vi "Teleop.vi"(10 "Match Info":T1={"Autonomous Elapsed Seconds"=0.0, "TeleOp Elapsed Seconds"=0.0, "Disabled Elapsed Seconds"=0.0, "Visited Autonomous"=FALSE, "Visited TeleOp"=FALSE, "Visited Disabled"=FALSE, "Autonomous Settings"={"Autonomous Style"=enum."Independent", "VI Refnum"=refnum}}, 11 "Call Context":T2) -> ()   [LabVIEW 2023]
doc: "This VI is called for each TeleOp packet received from the DS where the robot is not disabled. It is often used to read from the joysticks and update I/O or to update setpoints for timed control loops. It should complete and return within 20 milliseconds or it may miss DS packets."
uses:
  <vilib>/Rock Robotics/WPI/DriverStation/WPI_DriverStationDerivedRobotMode.ctl
  <vilib>/Rock Robotics/WPI/DriverStation/WPI_DriverStationMatch Info.ctl
  <vilib>/Rock Robotics/WPI/ThirdParty/Phoenix-LabVIEW/Motor Controller/Controls/CTRE_Phoenix_MotorControl_ControlMode.ctl
  <vilib>/Rock Robotics/WPI/Solenoid/WPI_SolenoidValue.ctl
  <vilib>/Rock Robotics/Network Tables/NT Read Boolean.vi
  <vilib>/Rock Robotics/Network Tables/NT Read Number.vi
  <vilib>/Rock Robotics/WPI/Utilities/WPI_GetSetVariantRefNum.vi
  <vilib>/Rock Robotics/Network Tables/NT Write Boolean Array.vi
  <vilib>/Rock Robotics/Network Tables/NT Write Numeric Array.vi
  Robot Global Data.vi
  <vilib>/Rock Robotics/WPI/ThirdParty/Phoenix-LabVIEW/Motor Controller/Get/CTRE_Phoenix_MotorController_GetSelectedSensorData.vi
  <vilib>/Rock Robotics/WPI/Solenoid/WPI_SolenoidSetEnum.vi
  <vilib>/Rock Robotics/WPI/ThirdParty/Phoenix-LabVIEW/Pigeon IMU/CTRE_PigeonIMU_GetAccumGyro.vi
  <vilib>/Rock Robotics/Network Tables/NT Write Number.vi
panel:
  out "Not Indexing and intaking":bool=TRUE
  out "Left Motor Encoder":i32
  out "Intake Output":dbl
  out "Sample Slider 0":dbl(slide) scale=0.0..5.0
  out "Sample Boolean 1":bool
  out "Sample Boolean 0":bool
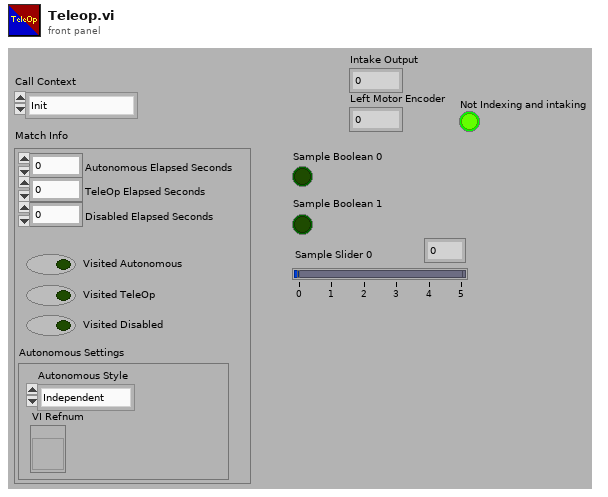
[diagram p1: front panel]
types:
  T1 = typedef "WPI_DriverStationMatch Info.ctl" = cluster{"Autonomous Elapsed Seconds":dbl, "TeleOp Elapsed Seconds":dbl, "Disabled Elapsed Seconds":dbl, "Visited Autonomous":bool, "Visited TeleOp":bool, "Visited Disabled":bool, "Autonomous Settings":cluster{"Autonomous Style":enum16{"Iterative", "Independent"}, "VI Refnum":refnum<vi>}}
  T2 = typedef "WPI_DriverStationDerivedRobotMode.ctl" = enum16{"Init", "Execute", "Stop"}
  T3 = typedef "WPI_SolenoidValue.ctl" = enum16{"Off", "On", "Forward", "Reverse"}
  T4 = typedef "CTRE_Phoenix_MotorControl_ControlMode.ctl" = u16
  T5 = typedef "WPI_JoystickDevRef.ctl" = cluster{"Device":T6}
  T6 = typedef "WPI_JoystickDeviceEnum.ctl" = enum16{"USB 0", "USB 1", "USB 2", "USB 3", "USB 4", "USB 5"}
  T7 = typedef "WPI_MotorControlDeviceRef.ctl" = cluster{"DeviceStatus":errorcluster, "Type":T8, "PWM":cluster{"PWM Channel":T9, "DeadBand":T10}, "CAN":cluster{"Device Number":u8, "SetOutput VI Ref":variant, "GetOutput VI Ref":variant, "Enable VI Ref":variant, "Disable VI Ref":variant, "Data":variant}, "Invert":bool, "DIO PWM":cluster{"PWM \"Enable\" Channel":T9, "DIOChannel":T11, "PWM Rate":dbl}}
  T8 = typedef "WPI_MotorControlType.ctl" = enum16{"PWM", "CAN", "DIO PWM"}
  T9 = typedef "FPGA_DIOPWMChannel.ctl" = enum8{"PWM 0", "PWM 1", "PWM 2", "PWM 3", "PWM 4", "PWM 5", "PWM 6", "PWM 7", "PWM 8", "PWM 9", "PWM MXP 0", "PWM MXP 1", "PWM MXP 2", "PWM MXP 3", "PWM MXP 4", "PWM MXP 5", "PWM MXP 6", "PWM MXP 7", "PWM MXP 8", "PWM MXP 9", "Invalid"}
  T10 = typedef "WPI_PWMDeadband.ctl" = cluster{"Name":string, "maxPositivePwm":i32, "minPositivePwm":i32, "centerPwm":i32, "maxNegativePwm":i32, "minNegativePwm":i32, "angularRange":u16}
  T11 = typedef "FPGA_DIOChannel.ctl" = enum8{"DIO 0", "DIO 1", "DIO 2", "DIO 3", "DIO 4", "DIO 5", "DIO 6", "DIO 7", "DIO 8", "DIO 9", "DIO MXP 0", "DIO MXP 1", "DIO MXP 2", "DIO MXP 3", "DIO MXP 4", "DIO MXP 5", "DIO MXP 6", "DIO MXP 7", "DIO MXP 8", "DIO MXP 9", "DIO MXP 10", "DIO MXP 11", "DIO MXP 12", "DIO MXP 13", "DIO MXP 14", "DIO MXP 15", "SPI Port CS1", "SPI Port CS2", "SPI Port CS3", "SPI Port MISO", "SPI Port MOSI", "Invalid"}
  T12 = typedef "WPI_RobotDriveDevRef.ctl" = cluster{"DevStatus":errorcluster, "Motors[]":T7[], "Square Inputs":bool, "Max Output":dbl}
  T13 = typedef "WPI_SolenoidDevRef.ctl" = cluster{"DevStatus":errorcluster, "Pneumatics Control Module":u8, "Forward Solenoid Channel":T14, "Reverse Solenoid Channel":T14}
  T14 = typedef "WPI_SolenoidChannel.ctl" = enum8{"Solenoid 0", "Solenoid 1", "Solenoid 2", "Solenoid 3", "Solenoid 4", "Solenoid 5", "Solenoid 6", "Solenoid 7", "Solenoid 8", "Solenoid 9", "Solenoid 10", "Solenoid 11", "Solenoid 12", "Solenoid 13", "Solenoid 14", "Solenoid 15", "Invalid"}
  T15 = typedef "WPI_ServoDeviceRef.ctl" = cluster{"DeviceStatus":errorcluster, "PWM Channel":T9, "DeadBand":T10}
  T16 = typedef "CTRE_PigeonIMU_DeviceRef.ctl" = cluster{"DeviceStatus":errorcluster, "Device Number":u8, "Type":T17, "Device ID":u32, "Handle":u64, "UsageFrame":u32, "Library Path":path}
  T17 = typedef "CTRE_PigeonIMU_ConnectionType.ctl" = u32
  T18 = typedef "WPI_SwitchDevRef.ctl" = cluster{"DevStatus":errorcluster, "DIO Channel":T11, "CntIndex":T19, "Normally Closed":bool}
  T19 = typedef "FPGA_CounterCtrSystemIndex.ctl" = enum8{"Ctr 0", "Ctr 1", "Ctr 2", "Ctr 3", "Ctr 4", "Ctr 5", "Ctr 6", "Ctr 7", "Invalid"}
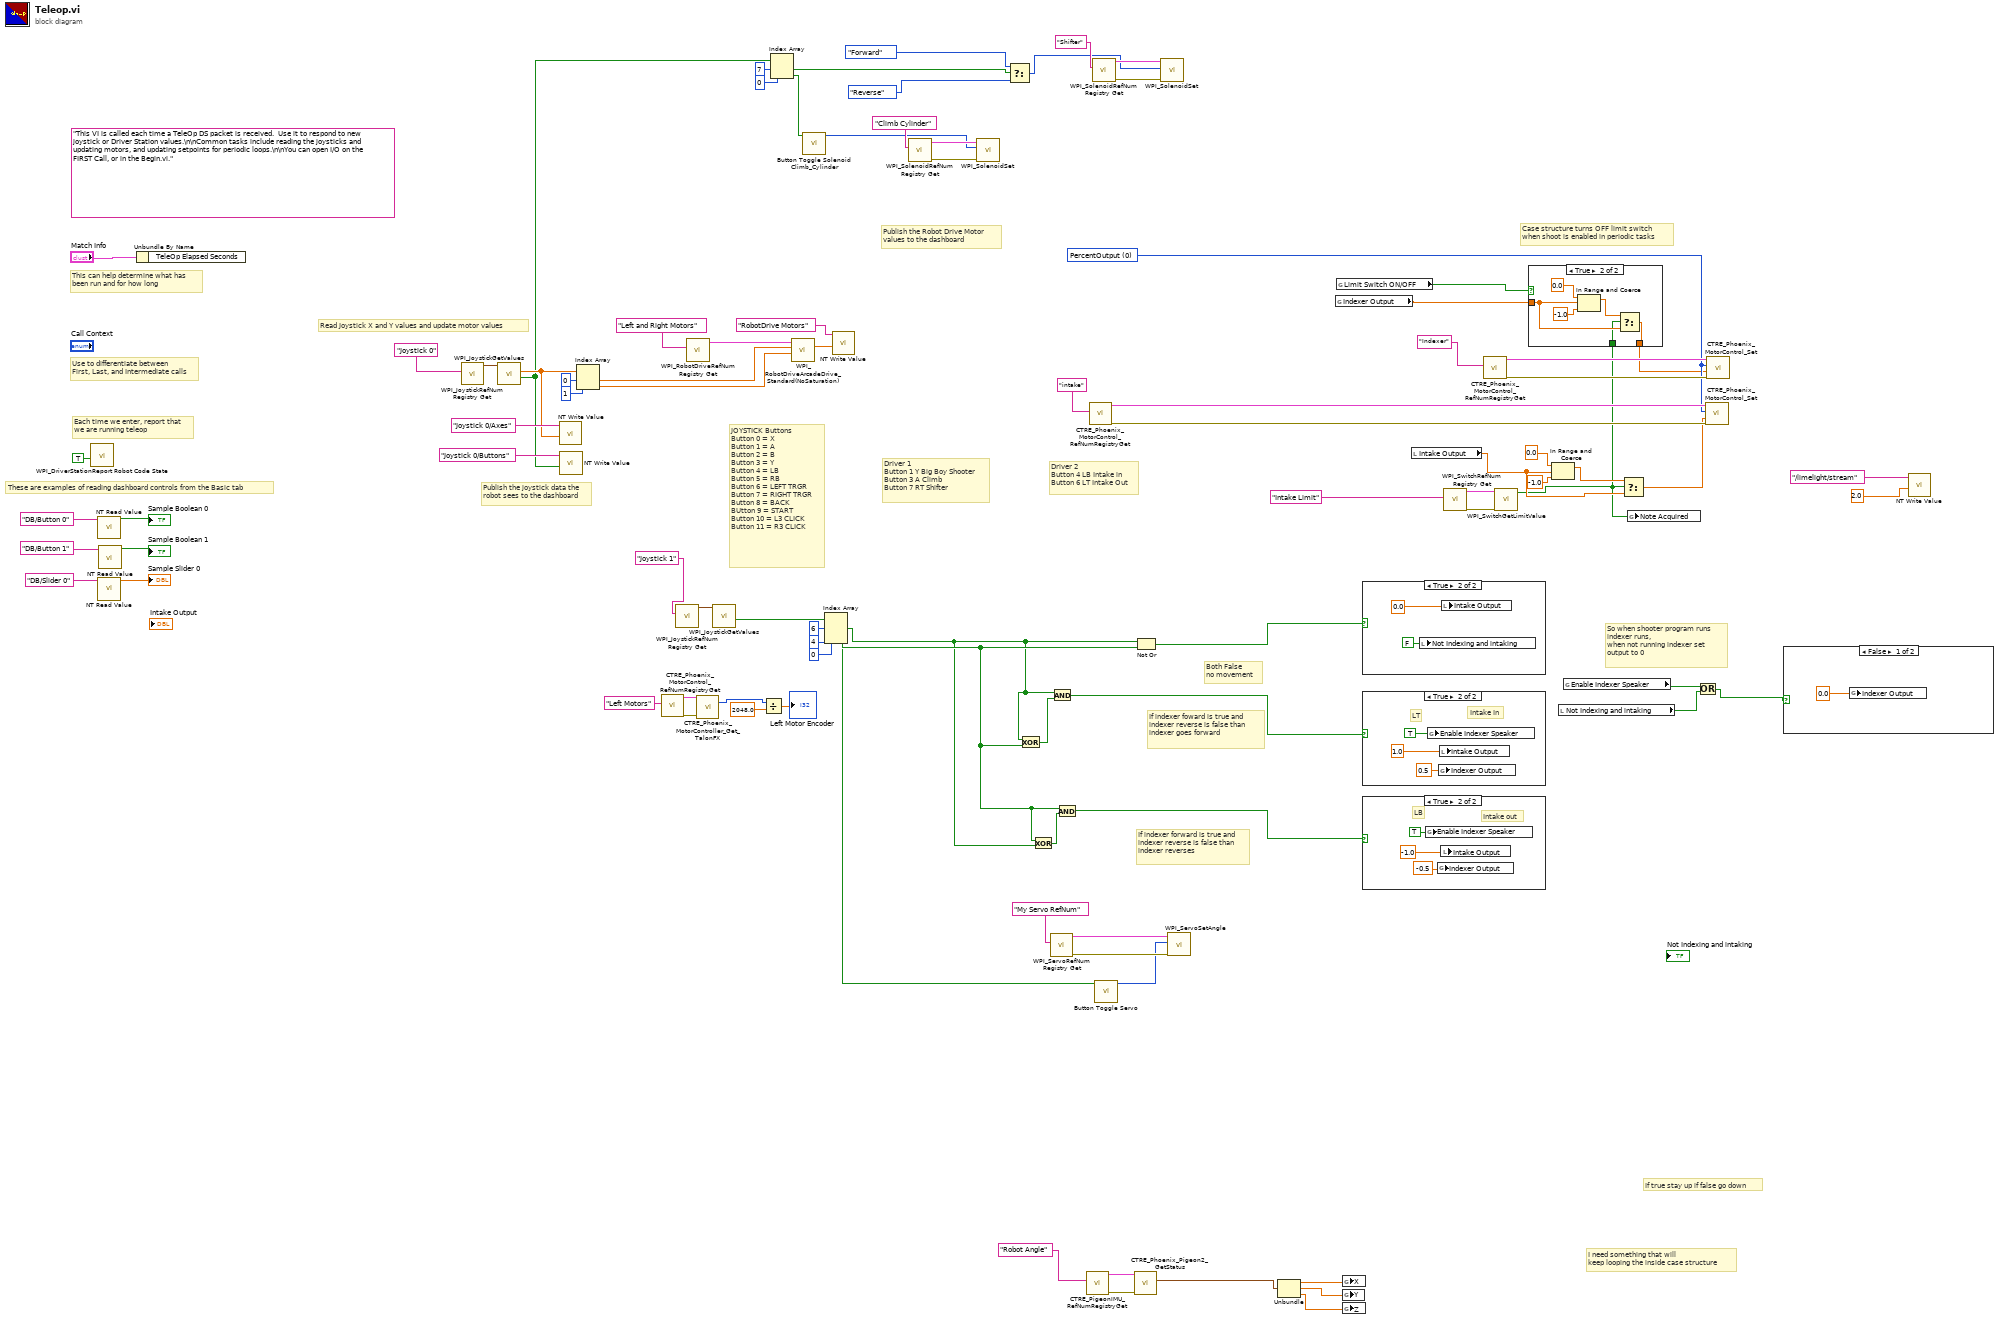
[diagram p0: block diagram]
diagram:
  w59 = T4 0 items=["PercentOutput"=0, "Position"=1, "Velocity"=2, "Current"=3, "Follower"=5, "MotionProfile"=6, "MotionMagic"=7, "MotionProfileArc"=10, "Disabled"=15] ("Control Mode")
  (unwired) "This VI is called each time a TeleOp DS packet is received.  Use it to respond to new joystick or Driver Station values.\n\nCommon tasks include reading the joysticks and updating motors, and updating setpoints for periodic loops.\n\nYou can open I/O on the FIRST Call, or in the Begin.vi."
  # "Driver 2\nButton 4 LB Intake in\nButton 6 LT Intake Out"
  # "Driver 1\nButton 1 Y Big Boy Shooter\nButton 3 A Climb\nButton 7 RT Shifter"
  # "I need something that will\nkeep looping the inside case structure"
  # "If true stay up if false go down"
  # "So when shooter program runs\nindexer runs,\nwhen not running indexer set\noutput to 0"
  # "Case structure turns OFF limit switch\nwhen shoot is enabled in periodic tasks"
  # "If indexer foward is true and\nindexer reverse is false than \nindexer goes forward"
  # "Both False\nno movement"
  # "If indexer forward is true and\nindexer reverse is false than \nindexer reverses"
  # "JOYSTICK Buttons\nButton 0 = X\nButton 1 = A\nButton 2 = B\nButton 3 = Y\nButton 4 = LB \nButton 5 = RB\nButton 6 = LEFT TRGR \nButton 7 = RIGHT TRGR \nButton 8 = BACK\nBUtton 9 = START\nButton 10 = L3 CLICK\nButton 11 = R3 CLICK"
  # "Publish the Robot Drive Motor\nvalues to the dashboard"
  # "Publish the joystick data the\nrobot sees to the dashboard"
  # "Read Joystick X and Y values and update motor values"
  # "These are examples of reading dashboard controls from the Basic tab"
  # "Each time we enter, report that\nwe are running teleop"
  # "Use to differentiate between\nFirst, Last, and Intermediate calls"
  # "This can help determine what has\nbeen run and for how long"
  n1 = call <vilib>:"WPI_DriverStationReport Robot Code State.vi"("TeleOp"=TRUE ("Autonomous")) -> ()  [unwired: 10 in, 1 out]
  n2 = call-poly <vilib>:"NT Read Value.vi"("name"="DB/Button 0" ("refnum name")) -> ("value"=→"Sample Boolean 0":bool)  [unwired: 8 in, 2 out]
  n3 = call-poly <vilib>:"NT Read Value.vi"("name"="DB/Slider 0" ("refnum name")) -> ("value"=→"Sample Slider 0":dbl)  [unwired: 8 in, 2 out]
  n4 = call-poly <vilib>:"NT Read Value.vi"("name"="DB/Button 1" ("refnum name")) -> ("value"=→"Sample Boolean 1":bool)  [unwired: 8 in, 2 out]
  n5 = Unbundle By Name("Match Info") -> ()  [unwired: 1 out]
  n6 = call <vilib>:"WPI_JoystickRefNum Registry Get.vi"("refnum name"="Joystick 0") -> ("JoystickDevRef"=w82:T5)  [unwired: 1 in, 9 out]
  n7 = call <vilib>:"WPI_JoystickGetValues.vi"("JoystickDevRef"=w82) -> ("Buttons"=w20:bool[], "Axes"=w79:dbl[])  [unwired: 6 in, 3 out]
  n8 = call-poly <vilib>:"NT Write Value.vi"("value"=w79, "name"="Joystick 0/Axes" ("Name")) -> ()  [unwired: 9 in, 1 out]
  n9 = call-poly <vilib>:"NT Write Value.vi"("value"=w20, "name"="Joystick 0/Buttons" ("Name")) -> ()  [unwired: 9 in, 1 out]
  n10 = Index Array(array=w79, index #1=0 ("index"), index #2=1 ("index")) -> (element #1=w73:dbl, element #2=w72:dbl)
  n11 = call <vilib>:"CTRE_Phoenix_MotorControl_RefNumRegistryGet.vi"("refnum name"="Left Motors") -> ("error out"=w47:errorcluster, "PhoenixMotorControlDevRef"=w48:T7)  [unwired: 9 in]
  n12 = call <vilib>:"WPI_JoystickRefNum Registry Get.vi"("refnum name"="Joystick 1") -> ("JoystickDevRef"=w18:T5)  [unwired: 1 in, 9 out]
  n13 = call <vilib>:"WPI_RobotDriveRefNum Registry Get.vi"("refnum name"="Left and Right Motors") -> ("RobotDriveDevRef"=w76:T12)  [unwired: 1 in, 9 out]
  n14 = call-poly <vilib>:"CTRE_Phoenix_MotorController_Get_TalonFX.vi"("PhoenixMotorControlDevRef"=w48, "error in"=w47) -> ("Position (Raw Sensor Units)"=w44:i32)  [unwired: 10 in, 3 out]
  n15 = call <vilib>:"WPI_JoystickGetValues.vi"("JoystickDevRef"=w18) -> ("Buttons"=w19:bool[])  [unwired: 6 in, 4 out]
  n16 = Divide(x=w44, y=2048.0) -> (x/y=→"Left Motor Encoder":dbl)
  n17 = Index Array(array=w20, index #1=7 ("index"), index #2=0 ("index")) -> (element #1=w33:bool, element #2=w31:bool)
  n18 = call <vilib>:"WPI_RobotDriveArcadeDrive_Standard(NoSaturation).vi"("Y axis value"=w72, "X axis value"=w73, "RobotDriveDevRef"=w76) -> ("Motor Values"=w75:dbl[])  [unwired: 1 in, 7 out]
  n19 = call "Button Toggle Solenoid Climb_Cylinder.vi"("Button A"=w31) -> ("Climb_Cylinder_Value"=w32:T3)  [unwired: 10 in]
  n20 = Index Array(array=w19, index #1=6 ("index"), index #2=4 ("index"), index #3=0 ("index")) -> (element #1=w13:bool, element #2=w14:bool, element #3=w6:bool)
  n21 = call-poly <vilib>:"NT Write Value.vi"("value"=w75, "name"="RobotDrive Motors" ("Name")) -> ()  [unwired: 9 in, 1 out]
  n22 = call <vilib>:"WPI_SolenoidRefNum Registry Get.vi"("refnum name"="Climb Cylinder") -> ("error out"=w36:errorcluster, "SolenoidDevRef"=w37:T13)  [unwired: 9 in]
  n23 = call-poly <vilib>:"WPI_SolenoidSet.vi"("error in (no error)"=w36, "Value"=w32, "SolenoidDevRef"=w37) -> ()  [unwired: 7 in, 2 out]
  n24 = Select(t=WPI_SolenoidValue."Forward" ("Value"), s=w33, f=WPI_SolenoidValue."Reverse" ("Value")) -> (s? t:f=w40:T3)
  n25 = Exclusive Or(1:w14, 2:w13) -> (0:w69:bool)
  n26 = Exclusive Or(1:w13, 2:w14) -> (0:w68:bool)
  n27 = call <vilib>:"WPI_ServoRefNum Registry Get.vi"("refnum name"="My Servo RefNum") -> ("error out"=w9:errorcluster, "ServoDeviceRef"=w8:T15)  [unwired: 9 in]
  n28 = And(x=w13, y=w69) -> (x .and. y?=w67:bool)
  n29 = And(x=w14, y=w68) -> (x .and. y?=w66:bool)
  n30 = call <vilib>:"CTRE_PigeonIMU_RefNumRegistryGet.vi"("refnum name"="Robot Angle") -> ("error out"=w28:errorcluster, "PigeonIMUDevRef"=w27:T16)  [unwired: 9 in]
  n31 = call <vilib>:"CTRE_Phoenix_MotorControl_RefNumRegistryGet.vi"("refnum name"="intake") -> ("error out"=w63:errorcluster, "PhoenixMotorControlDevRef"=w64:T7)  [unwired: 9 in]
  n32 = call <vilib>:"WPI_SolenoidRefNum Registry Get.vi"("refnum name"="Shifter") -> ("error out"=w42:errorcluster, "SolenoidDevRef"=w41:T13)  [unwired: 9 in]
  n33 = call "Button Toggle Servo.vi"("Boolean"=w6) -> ("Camera Angle"=w5:i32)  [unwired: 10 in]
  n34 = call-poly <vilib>:"CTRE_Phoenix_Pigeon2_GetStatus.vi"("error in (no error)"=w28, "PigeonIMUDevRef"=w27) -> ("AccumGyro"=w29:cluster{"X":dbl, "Y":dbl, "Z":dbl})  [unwired: 7 in, 2 out]
  n35 = Not Or(1:w14, 2:w13) -> (0:w65:bool)
  n36 = call-poly <vilib>:"WPI_SolenoidSet.vi"("error in (no error)"=w42, "Value"=w40, "SolenoidDevRef"=w41) -> ()  [unwired: 7 in, 2 out]
  n37 = call <vilib>:"WPI_ServoSetAngle.vi"("error in (no error)"=w9, "Angle"=w5, "ServoDeviceRef"=w8) -> ()  [unwired: 7 in, 2 out]
  n38 = Unbundle(w29) -> ("X"=w23:dbl, "Y"=w22:dbl, "Z"=w21:dbl)
  n39 = global read "Robot Global Data.vi" "Indexer Output"() -> (w24:dbl)
  n40 = global read "Robot Global Data.vi" "Limit Switch ON/OFF"() -> (w25:bool)
  n41 = global write "Robot Global Data.vi" "X"(w23) -> ()
  n42 = global write "Robot Global Data.vi" "Y"(w22) -> ()
  n43 = global write "Robot Global Data.vi" "Z"(w21) -> ()
  n44 = case shown="True" w65 {
    frame False {
    }
    frame True {
      n45 = local write "Not Indexing and intaking"(FALSE ("Not Indexing and intaking")) -> ()
      n46 = local write "Intake Output"(0.0) -> ()
    }
  }
  n47 = case shown="True" w67 {
    frame False {
    }
    frame True {
      # "Intake In"
      # "LT"
      n48 = global write "Robot Global Data.vi" "Enable Indexer Speaker"(TRUE ("Enable Indexer")) -> ()
      n49 = global write "Robot Global Data.vi" "Indexer Output"(0.5 ("Indexer Output")) -> ()
      n50 = local write "Intake Output"(1.0) -> ()
    }
  }
  n51 = case shown="True" w66 {
    frame False {
    }
    frame True {
      # "Intake out"
      # "LB"
      n52 = global write "Robot Global Data.vi" "Enable Indexer Speaker"(TRUE ("Enable Indexer")) -> ()
      n53 = global write "Robot Global Data.vi" "Indexer Output"(-0.5 ("Indexer Output")) -> ()
      n54 = local write "Intake Output"(-1.0) -> ()
    }
  }
  n55 = local read "Intake Output"() -> (w58:dbl)
  n56 = call <vilib>:"WPI_SwitchRefNum Registry Get.vi"("refnum name"="Intake Limit") -> ("error out"=w57:errorcluster, "SwitchDevRef"=w54:T18)  [unwired: 9 in]
  n57 = call <vilib>:"CTRE_Phoenix_MotorControl_RefNumRegistryGet.vi"("refnum name"="Indexer") -> ("error out"=w60:errorcluster, "PhoenixMotorControlDevRef"=w61:T7)  [unwired: 9 in]
  n58 = call <vilib>:"WPI_SwitchGetLimitValue.vi"("error in (no error)"=w57, "SwitchDevRef"=w54) -> ("Switch Pressed"=w3:bool)  [unwired: 7 in, 2 out]
  n59 = case shown="True" w25 {
    tunnel: w3 -> [_ w101]
    tunnel: [w100 w102] -> w50
    tunnel: w24 -> [w100 w103]
    frame False {
    }
    frame True {
      n60 = In Range and Coerce(upper limit=0.0, x=w103, lower limit=-1.0) -> (coerced(x)=w106:dbl)  [unwired: 1 out]
      n61 = Select(t=w106, s=w101, f=w103) -> (s? t:f=w102:dbl)
    }
  }
  n62 = In Range and Coerce(upper limit=0.0, x=w58, lower limit=-1.0) -> (coerced(x)=w55:dbl)  [unwired: 1 out]
  n63 = local read "Not Indexing and intaking"() -> (w11:bool)
  n64 = global read "Robot Global Data.vi" "Enable Indexer Speaker"() -> (w12:bool)
  n65 = Select(t=w55, s=w3, f=w58) -> (s? t:f=w51:dbl)
  n66 = global write "Robot Global Data.vi" "Note Acquired"(w3) -> ()
  n67 = Or(x=w12, y=w11) -> (x .or. y?=w4:bool)
  n68 = call <vilib>:"CTRE_Phoenix_MotorControl_Set.vi"("error in (no error)"=w63, "Output"=w51, "Control Mode"=w59, "PhoenixMotorControlDevRef"=w64) -> ()  [unwired: 6 in, 2 out]
  n69 = call <vilib>:"CTRE_Phoenix_MotorControl_Set.vi"("error in (no error)"=w60, "Output"=w50, "Control Mode"=w59, "PhoenixMotorControlDevRef"=w61) -> ()  [unwired: 6 in, 2 out]
  n70 = case shown="False" w4 {
    frame False {
      n71 = global write "Robot Global Data.vi" "Indexer Output"(0.0) -> ()
    }
    frame True {
    }
  }
  n72 = call-poly <vilib>:"NT Write Value.vi"("value"=2.0, "name"="/limelight/stream" ("Name")) -> ()  [unwired: 9 in, 1 out]
